vi "emi_Wait for S&E Message.vi"(7 "timeout in ms (5)":i32=5, 11 "error in (no error)":errorcluster) -> (4 "timed out?":bool, 8 "E&S Message":T1, 15 "error out":errorcluster)   [LabVIEW 2011]
doc: "Wait for S&E Message.\nIf error in, this vi will wait 1 ms, befor continuing(to avoid spinning loops"
uses:
  Private/_emi_ S&E Message.ctl
  Private/_emi_ S&E Message type.ctl
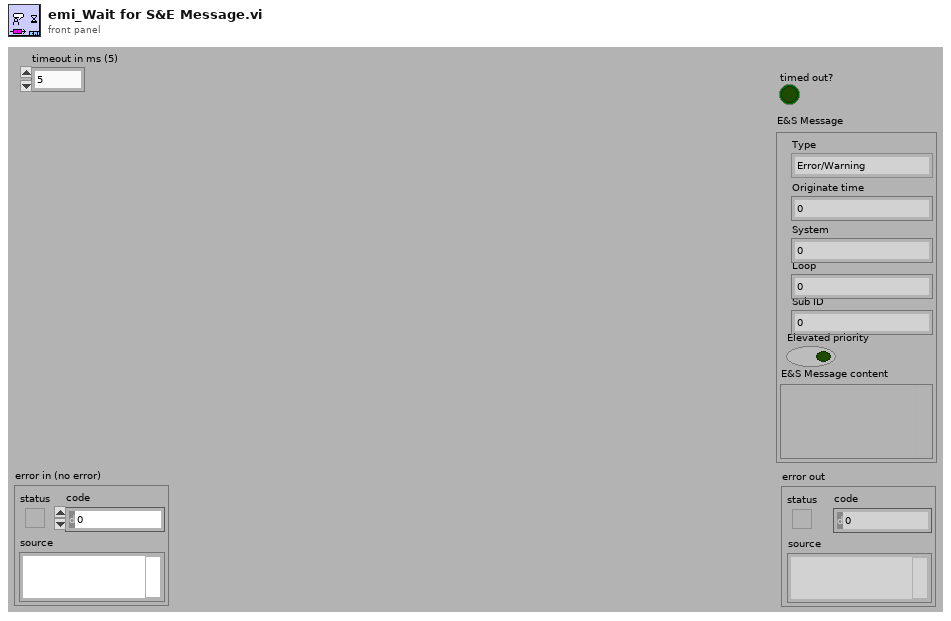
[diagram p1: front panel]
types:
  T1 = typedef "_emi_ S&E Message.ctl" = cluster{"Type":T2, "Originate time":dbl, "System":u8, "Loop":u16, "Sub ID":u16, "Elevated priority":bool, "E&S Message content":variant}
  T2 = typedef "_emi_ S&E Message type.ctl" = enum16{"Error/Warning", "Note", "Debug", "Event", "Alarm Analog", "Alarm Digital", "Annotation"}
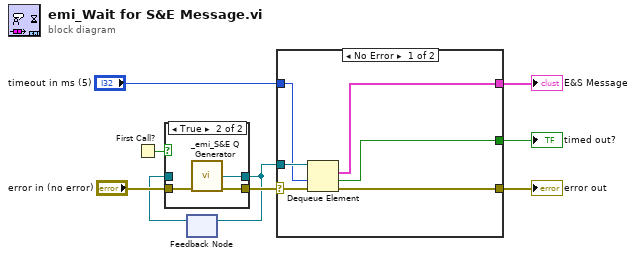
[diagram p0: block diagram]
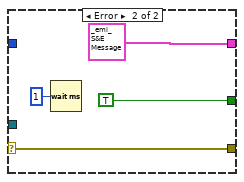
[diagram p3: hidden frame]
diagram:
  n1 = First Call?() -> (First Call?: T/F=w5:bool)
  n2 = feedback #1() -> (w6:refnum<queue>)  [unwired: 1 in]
  n3 = case shown="True" w5 {
    tunnel: "error in (no error)" -> [w10 w14]
    tunnel: [w10 w13] -> w7
    tunnel: [w11 w12] -> w4
    tunnel: w6 -> [w11 _]
    frame False {
    }
    frame True {
      n4 = call "_emi_S&E Q Generator.vi"("error in (no error)"=w14) -> ("E&S Message Q"=w12:refnum<queue>, "error out"=w13:errorcluster)  [unwired: 13 in]
    }
  }
  n5 = feedback-in #1(w4) -> ()
  n6 = case shown="No Error" w7 {
    selector: w7 -> [w20 w24]
    tunnel: [w19 w24] -> w9
    tunnel: w4 -> [w18 _]
    tunnel: "timeout in ms (5)" -> [w17 _]
    tunnel: [w16 TRUE ("timed out?")] -> w2
    tunnel: [w15 T1 {"Type"=enum."Error/Warning", "Originate time"=0.0, "System"=0, "Loop"=0, "Sub ID"=0, "Elevated priority"=FALSE, "E&S Message content"=variant} ("E&S Message")] -> w1
    frame No Error {
      n7 = Dequeue Element(queue=w18, timeout in ms (-1)=w17, error in (no error)=w20) -> (element=w15:T1, timed out?=w16:bool, error out=w19:errorcluster)  [unwired: 1 out]
    }
    frame Error {
      n8 = Wait (ms)(milliseconds to wait=u32 1) -> ()  [unwired: 1 out]
    }
  }
  "error out" <- w9
  "timed out?" <- w2
  "E&S Message" <- w1
